vi "Submit.vi"(0 "NSIS Installer In":refnum<class "NSIS Installer.lvclass">) -> (4 "NSIS Installer Out":refnum<class "NSIS Installer.lvclass">)   [LabVIEW 2017, in "CL_G3_VIComponentBuilder.lvlib" / "NSIS Installer.lvclass"]
doc: "Invokes the commit behaivor specified by this export and any additional operations deemed necessary by the export."
uses:
  NSIS Installer.lvclass
  C:/Tool Chain Support/Software Module Builder/Source/Exports/Exports/Export.lvclass
  Exports/Export.lvclass/Export.ctl
  Exports/Accessors/Write Export Operation Errors.vi
  Exports/Accessors/Read Commit behavior.vi
  Exports/Accessors/Read Exported Build Specification Path.vi
  Exports/Accessors/Read Export Build Specification.vi
  Exports/Accessors/Read Export Operation Errors.vi
  Compound Installer/Compound_Installer.lvclass
  Commit Behavior/Commit/Commit.lvclass
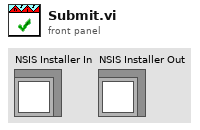
[diagram p1: front panel]
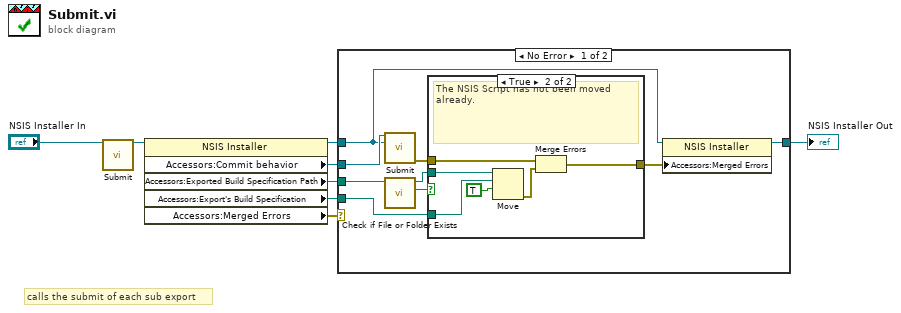
[diagram p0: block diagram]
diagram:
  # "calls the submit of each sub export"
  n1 = call-parent "Submit.vi"("Compound_Installer In"="NSIS Installer In") -> ("Compound_Installer Out"=w2:refnum<class "NSIS Installer.lvclass">)  [unwired: 14 in]
  n2 = property class="NSIS Installer"(reference=w2) -> (reference out=w7:refnum<class "NSIS Installer.lvclass">, "Accessors:Commit behavior"=w8:refnum<class "Commit.lvclass">, "Accessors:Exported Build Specification Path"=w5:path, "Accessors:Export's Build Specification"=w6:path, "Accessors:Merged Errors"=w4:errorcluster)  [unwired: 1 in, 1 out]
  n3 = case shown="No Error" w4 {
    tunnel: w8 -> [w17 _]
    tunnel: w7 -> [w16 w25]
    tunnel: w6 -> [w15 _]
    tunnel: w5 -> [w12 _]
    tunnel: [w9 w25] -> w1
    frame No Error {
      n4 = call-dynamic "Submit.vi"("Commit in"=w17, "Export"=w16) -> ("error out"=w14:errorcluster)  [unwired: 12 in, 1 out]
      n5 = call <vilib>:"Check if File or Folder Exists.vi"("path"=w12) -> ("file or folder exists?"=w10:bool, "dup path"=w11:path)  [unwired: 8 in, 1 out]
      n6 = case shown="True" w10 {
        tunnel: w15 -> [_ w23]
        tunnel: w14 -> [w18 w22]
        tunnel: [w18 w20] -> w13
        tunnel: w11 -> [_ w19]
        frame False {
          # "The NSIS Script was already moved as a result of the the installer owning multiple exports."
        }
        frame True {
          # "The NSIS Script has not been moved already."
          n7 = Move(source path=w19, 9:TRUE ("overwrite (F)"), 10:w23) -> (error out=w21:errorcluster)  [unwired: 2 in, 2 out]
          n8 = Merge Errors(w22, w21) -> (w20:errorcluster)
        }
      }
      n9 = property class="NSIS Installer"(reference=w16, "Accessors:Merged Errors"=w13) -> (reference out=w9:refnum<class "NSIS Installer.lvclass">)  [unwired: 1 in, 1 out]
    }
    frame Error {
    }
  }
  "NSIS Installer Out" <- w1
